vi "Extract subclasses from Pressure device.vi"(9 "Data In":string, 10 "Class":string, 11 "Pressure Device Settings in":T1) -> (1 "Data out":string, 3 "Pressure Device Settings out":T1)   [LabVIEW 2014, in "Mercury iXX.lvlib" / "Pressure.lvlib"]
uses:
  Pressure.lvlib
  Program Files (x86)/National Instruments/LabVIEW 2014/Public/Libraries/Pressure/Controls/Pressure Device (Read).ctl
  Controls/Manufacturing Data.ctl
  Controls/Pressure Sensor Type.ctl
  Controls/Calibration Cluster.ctl
  Controls/Calibration Interpolation.ctl
  Controls/Loop Cluster.ctl
  Controls/Pressure Signals Cluster.ctl
  Mercury iXX.lvlib
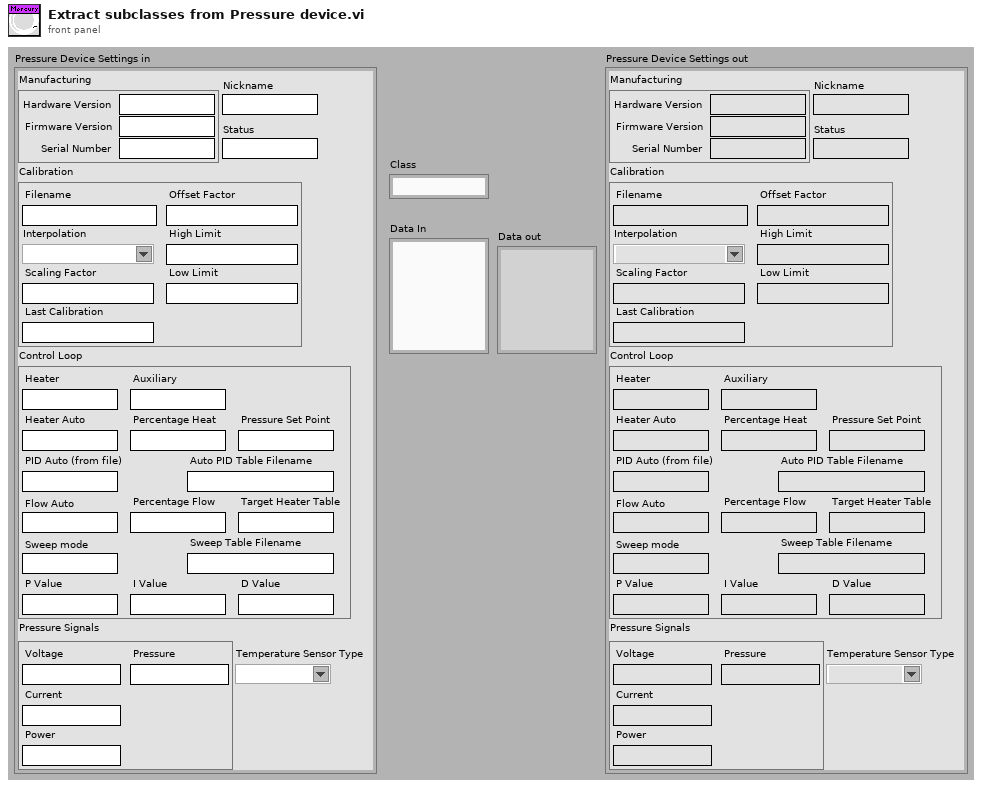
[diagram p1: front panel]
types:
  T1 = typedef "Mercury iXX.lvlib/Pressure.lvlib/Pressure Device (Read).ctl" = cluster{"Manufacturing":T2, "Temperature Sensor Type":T3, "Calibration":T4, "Control Loop":T6, "Pressure Signals":T7, "Nickname":string, "Status":string}
  T2 = typedef "Mercury iXX.lvlib/Manufacturing Data.ctl" = cluster{"Hardware Version":string, "Firmware Version":string, "Serial Number":string}
  T3 = typedef "Mercury iXX.lvlib/Pressure.lvlib/Pressure Sensor Type.ctl" = string
  T4 = typedef "Mercury iXX.lvlib/Pressure.lvlib/Calibration Cluster.ctl" = cluster{"Filename":string, "Interpolation":T5, "Scaling Factor":string, "Offset Factor":string, "High Limit":string, "Low Limit":string, "Last Calibration":string}
  T5 = typedef "Mercury iXX.lvlib/Pressure.lvlib/Calibration Interpolation.ctl" = string
  T6 = typedef "Mercury iXX.lvlib/Pressure.lvlib/Loop Cluster.ctl" = cluster{"Heater":string, "Auxiliary":string, "Heater Auto":string, "Percentage Heat":string, "Pressure Set Point":string, "PID Auto (from file)":string, "P Value":string, "I Value":string, "D Value":string, "Auto PID Table Filename":string, "Flow Auto":string, "Target Heater Table":string, "Sweep mode":string, "Sweep Table Filename":string, "Percentage Flow":string}
  T7 = typedef "Mercury iXX.lvlib/Pressure.lvlib/Pressure Signals Cluster.ctl" = cluster{"Voltage":string, "Current":string, "Power":string, "Pressure":string}
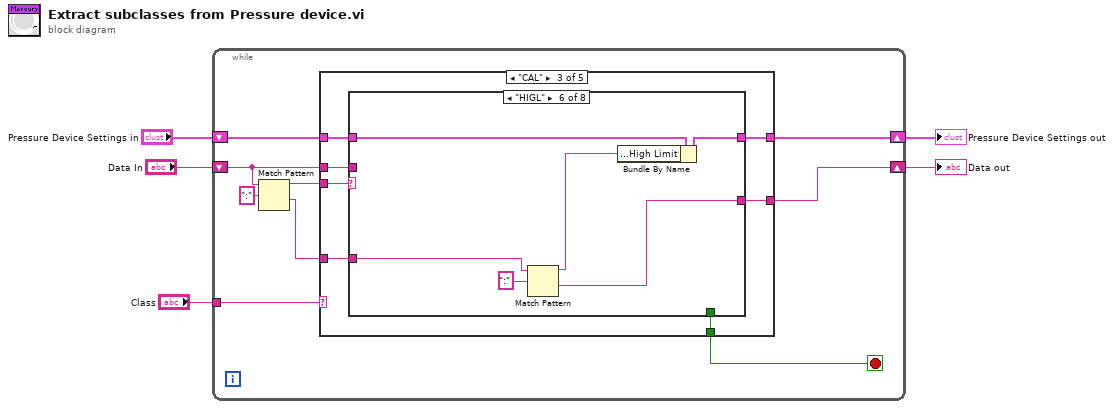
[diagram p0: block diagram]
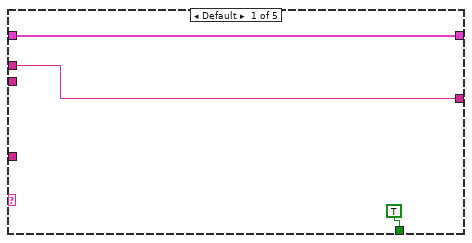
[diagram p2: hidden frame]
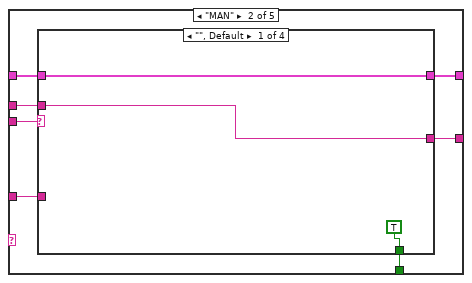
[diagram p3: hidden frame]
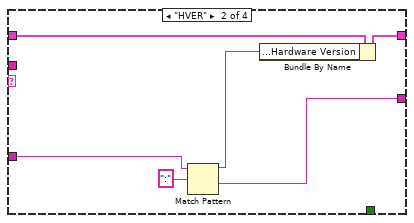
[diagram p4: hidden frame]
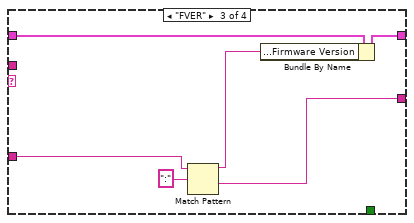
[diagram p5: hidden frame]
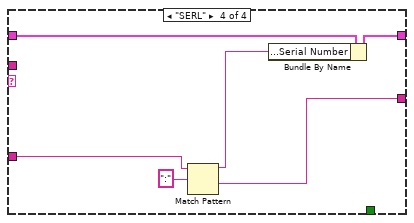
[diagram p6: hidden frame]
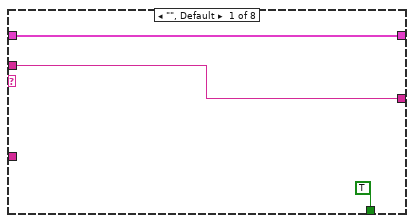
[diagram p7: hidden frame]
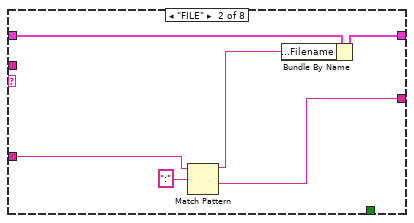
[diagram p8: hidden frame]
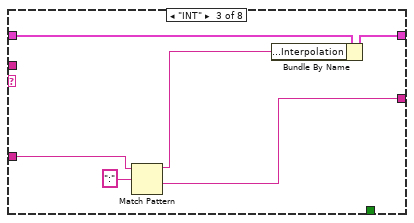
[diagram p9: hidden frame]
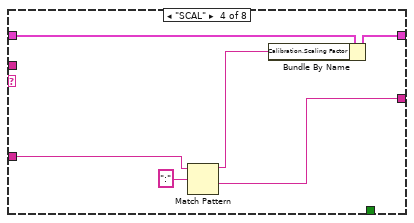
[diagram p10: hidden frame]
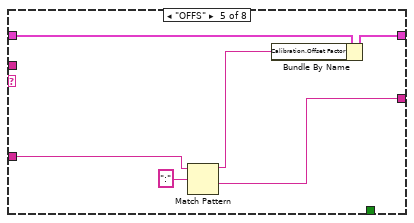
[diagram p11: hidden frame]
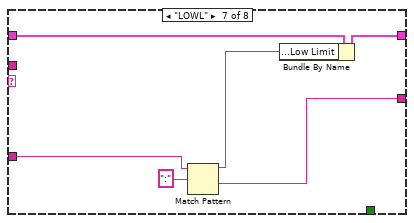
[diagram p12: hidden frame]
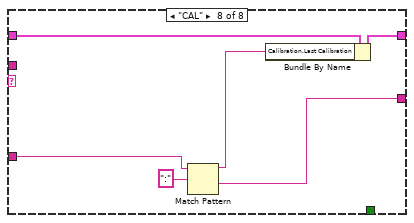
[diagram p13: hidden frame]
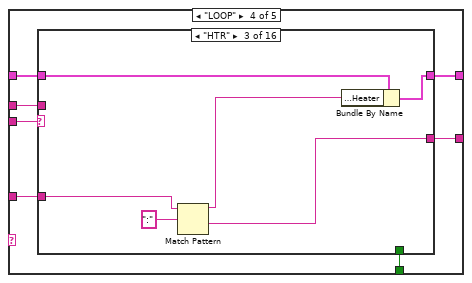
[diagram p14: hidden frame]
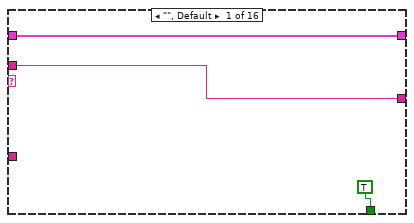
[diagram p15: hidden frame]
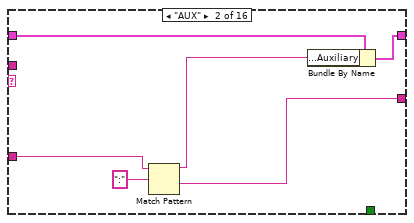
[diagram p16: hidden frame]
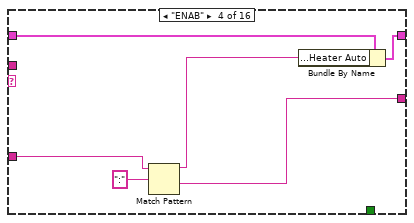
[diagram p17: hidden frame]
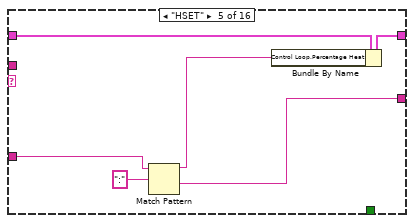
[diagram p18: hidden frame]
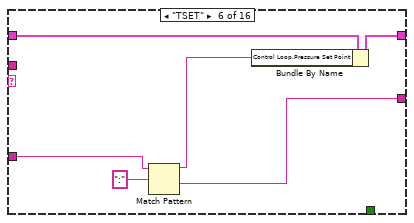
[diagram p19: hidden frame]
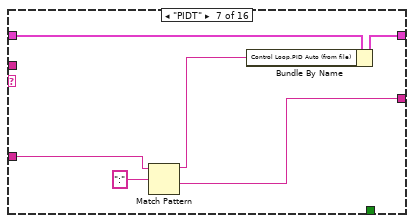
[diagram p20: hidden frame]
diagram:
  n1 = while {
    tunnel: "Class" -> [w7]
    shift-right: [w10] -> w4
    shift-left: "Data In" -> [w8]
    shift-right: [w12] -> w3
    shift-left: "Pressure Device Settings in" -> [w13]
    stop <- w6 stop-if-true
    n2 = Match Pattern(string=w8, regular expression=":") -> (before substring=w9:string, after substring=w11:string)  [unwired: 3 out]
    n3 = case shown="\"CAL\"" w7 {
      tunnel: w13 -> [w17 w24 w52 w104 w204]
      tunnel: [w17 w23 w51 w103 w203] -> w12
      tunnel: w11 -> [_ w22 w50 w102 w202]
      tunnel: [w16 w21 w49 w101 w201] -> w10
      tunnel: w9 -> [_ w20 w48 w100 w200]
      tunnel: w8 -> [w16 w19 w47 w99 w199]
      tunnel: [TRUE w18 w46 w98 w198] -> w6
      frame Default {
      }
      frame "MAN" {
        n4 = case shown="\"\", Default" w20 {
          tunnel: w24 -> [w27 w33 w39 w45]
          tunnel: [w27 w32 w38 w44] -> w23
          tunnel: w22 -> [_ w31 w37 w43]
          tunnel: [w26 w30 w36 w42] -> w21
          tunnel: w19 -> [w26 _ _ _]
          tunnel: [TRUE _ _ _] -> w18
          frame "", Default {
          }
          frame "HVER" {
            n5 = Match Pattern(string=w31, regular expression=":") -> (before substring=w28:string, after substring=w30:string)  [unwired: 3 out]
            n6 = Bundle By Name(cluster=w33, "Manufacturing.Hardware Version"=w28) -> (w32:T1)
          }
          frame "FVER" {
            n7 = Match Pattern(string=w37, regular expression=":") -> (before substring=w34:string, after substring=w36:string)  [unwired: 3 out]
            n8 = Bundle By Name(cluster=w39, "Manufacturing.Firmware Version"=w34) -> (w38:T1)
          }
          frame "SERL" {
            n9 = Match Pattern(string=w43, regular expression=":") -> (before substring=w40:string, after substring=w42:string)  [unwired: 3 out]
            n10 = Bundle By Name(cluster=w45, "Manufacturing.Serial Number"=w40) -> (w44:T1)
          }
        }
      }
      frame "CAL" {
        n11 = case shown="\"HIGL\"" w48 {
          tunnel: w52 -> [w55 w61 w67 w73 w79 w85 w91 w97]
          tunnel: [w55 w60 w66 w72 w78 w84 w90 w96] -> w51
          tunnel: w50 -> [_ w59 w65 w71 w77 w83 w89 w95]
          tunnel: [w54 w58 w64 w70 w76 w82 w88 w94] -> w49
          tunnel: w47 -> [w54 _ _ _ _ _ _ _]
          tunnel: [TRUE _ _ _ _ _ _ _] -> w46
          frame "", Default {
          }
          frame "FILE" {
            n12 = Match Pattern(string=w59, regular expression=":") -> (before substring=w56:string, after substring=w58:string)  [unwired: 3 out]
            n13 = Bundle By Name(cluster=w61, "Calibration.Filename"=w56) -> (w60:T1)
          }
          frame "INT" {
            n14 = Match Pattern(string=w65, regular expression=":") -> (before substring=w62:string, after substring=w64:string)  [unwired: 3 out]
            n15 = Bundle By Name(cluster=w67, "Calibration.Interpolation"=w62) -> (w66:T1)
          }
          frame "SCAL" {
            n16 = Match Pattern(string=w71, regular expression=":") -> (before substring=w68:string, after substring=w70:string)  [unwired: 3 out]
            n17 = Bundle By Name(cluster=w73, "Calibration.Scaling Factor"=w68) -> (w72:T1)
          }
          frame "OFFS" {
            n18 = Match Pattern(string=w77, regular expression=":") -> (before substring=w74:string, after substring=w76:string)  [unwired: 3 out]
            n19 = Bundle By Name(cluster=w79, "Calibration.Offset Factor"=w74) -> (w78:T1)
          }
          frame "HIGL" {
            n20 = Match Pattern(string=w83, regular expression=":") -> (before substring=w80:string, after substring=w82:string)  [unwired: 3 out]
            n21 = Bundle By Name(cluster=w85, "Calibration.High Limit"=w80) -> (w84:T1)
          }
          frame "LOWL" {
            n22 = Match Pattern(string=w89, regular expression=":") -> (before substring=w86:string, after substring=w88:string)  [unwired: 3 out]
            n23 = Bundle By Name(cluster=w91, "Calibration.Low Limit"=w86) -> (w90:T1)
          }
          frame "CAL" {
            n24 = Match Pattern(string=w95, regular expression=":") -> (before substring=w92:string, after substring=w94:string)  [unwired: 3 out]
            n25 = Bundle By Name(cluster=w97, "Calibration.Last Calibration"=w92) -> (w96:T1)
          }
        }
      }
      frame "LOOP" {
        n26 = case shown="\"HTR\"" w100 {
          tunnel: w104 -> [w107 w113 w119 w125 w131 w137 w143 w149 w155 w161 w167 w173 w179 w185 w191 w197]
          tunnel: [w107 w112 w118 w124 w130 w136 w142 w148 w154 w160 w166 w172 w178 w184 w190 w196] -> w103
          tunnel: w102 -> [_ w110 w116 w122 w128 w134 w140 w146 w153 w159 w165 w171 w177 w183 w189 w195]
          tunnel: [w106 w109 w115 w121 w127 w133 w139 w145 w152 w158 w164 w170 w176 w182 w188 w194] -> w101
          tunnel: w99 -> [w106 _ _ _ _ _ _ _ _ _ _ _ _ _ _ _]
          tunnel: [TRUE _ _ _ _ _ _ _ _ _ _ _ _ _ _ _] -> w98
          frame "", Default {
          }
          frame "AUX" {
            n27 = Match Pattern(string=w110, regular expression=":") -> (before substring=w108:string, after substring=w109:string)  [unwired: 3 out]
            n28 = Bundle By Name(cluster=w113, "Control Loop.Auxiliary"=w108) -> (w112:T1)
          }
          frame "HTR" {
            n29 = Match Pattern(string=w116, regular expression=":") -> (before substring=w114:string, after substring=w115:string)  [unwired: 3 out]
            n30 = Bundle By Name(cluster=w119, "Control Loop.Heater"=w114) -> (w118:T1)
          }
          frame "ENAB" {
            n31 = Match Pattern(string=w122, regular expression=":") -> (before substring=w120:string, after substring=w121:string)  [unwired: 3 out]
            n32 = Bundle By Name(cluster=w125, "Control Loop.Heater Auto"=w120) -> (w124:T1)
          }
          frame "HSET" {
            n33 = Match Pattern(string=w128, regular expression=":") -> (before substring=w126:string, after substring=w127:string)  [unwired: 3 out]
            n34 = Bundle By Name(cluster=w131, "Control Loop.Percentage Heat"=w126) -> (w130:T1)
          }
          frame "TSET" {
            n35 = Match Pattern(string=w134, regular expression=":") -> (before substring=w132:string, after substring=w133:string)  [unwired: 3 out]
            n36 = Bundle By Name(cluster=w137, "Control Loop.Pressure Set Point"=w132) -> (w136:T1)
          }
          frame "PIDT" {
            n37 = Match Pattern(string=w140, regular expression=":") -> (before substring=w138:string, after substring=w139:string)  [unwired: 3 out]
            n38 = Bundle By Name(cluster=w143, "Control Loop.PID Auto (from file)"=w138) -> (w142:T1)
          }
          frame "PIDF" {
            n39 = Match Pattern(string=w146, regular expression=":") -> (before substring=w144:string, after substring=w145:string)  [unwired: 3 out]
            n40 = Bundle By Name(cluster=w149, "Control Loop.Auto PID Table Filename"=w144) -> (w148:T1)
          }
          frame "P" {
            n41 = Match Pattern(string=w153, regular expression=":") -> (before substring=w150:string, after substring=w152:string)  [unwired: 3 out]
            n42 = Bundle By Name(cluster=w155, "Control Loop.P Value"=w150) -> (w154:T1)
          }
          frame "I" {
            n43 = Match Pattern(string=w159, regular expression=":") -> (before substring=w156:string, after substring=w158:string)  [unwired: 3 out]
            n44 = Bundle By Name(cluster=w161, "Control Loop.I Value"=w156) -> (w160:T1)
          }
          frame "D" {
            n45 = Match Pattern(string=w165, regular expression=":") -> (before substring=w162:string, after substring=w164:string)  [unwired: 3 out]
            n46 = Bundle By Name(cluster=w167, "Control Loop.D Value"=w162) -> (w166:T1)
          }
          frame "FAUT" {
            n47 = Match Pattern(string=w171, regular expression=":") -> (before substring=w168:string, after substring=w170:string)  [unwired: 3 out]
            n48 = Bundle By Name(cluster=w173, "Control Loop.Flow Auto"=w168) -> (w172:T1)
          }
          frame "FSET" {
            n49 = Match Pattern(string=w177, regular expression=":") -> (before substring=w174:string, after substring=w176:string)  [unwired: 3 out]
            n50 = Bundle By Name(cluster=w179, "Control Loop.Percentage Flow"=w174) -> (w178:T1)
          }
          frame "THTF" {
            n51 = Match Pattern(string=w183, regular expression=":") -> (before substring=w180:string, after substring=w182:string)  [unwired: 3 out]
            n52 = Bundle By Name(cluster=w185, "Control Loop.Target Heater Table"=w180) -> (w184:T1)
          }
          frame "SWMD" {
            n53 = Match Pattern(string=w189, regular expression=":") -> (before substring=w186:string, after substring=w188:string)  [unwired: 3 out]
            n54 = Bundle By Name(cluster=w191, "Control Loop.Sweep mode"=w186) -> (w190:T1)
          }
          frame "SWFL" {
            n55 = Match Pattern(string=w195, regular expression=":") -> (before substring=w192:string, after substring=w194:string)  [unwired: 3 out]
            n56 = Bundle By Name(cluster=w197, "Control Loop.Sweep Table Filename"=w192) -> (w196:T1)
          }
        }
      }
      frame "SIG" {
        n57 = case shown="\"PRES\"" w200 {
          tunnel: w204 -> [w207 w213 w219 w225 w231]
          tunnel: [w207 w212 w218 w224 w230] -> w203
          tunnel: w202 -> [_ w211 w217 w223 w229]
          tunnel: [w206 w210 w216 w222 w228] -> w201
          tunnel: w199 -> [w206 _ _ _ _]
          tunnel: [TRUE _ _ _ _] -> w198
          frame "", Default {
          }
          frame "VOLT" {
            n58 = Match Pattern(string=w211, regular expression=":") -> (before substring=w208:string, after substring=w210:string)  [unwired: 3 out]
            n59 = Bundle By Name(cluster=w213, "Pressure Signals.Voltage"=w208) -> (w212:T1)
          }
          frame "CURR" {
            n60 = Match Pattern(string=w217, regular expression=":") -> (before substring=w214:string, after substring=w216:string)  [unwired: 3 out]
            n61 = Bundle By Name(cluster=w219, "Pressure Signals.Current"=w214) -> (w218:T1)
          }
          frame "POWR" {
            n62 = Match Pattern(string=w223, regular expression=":") -> (before substring=w220:string, after substring=w222:string)  [unwired: 3 out]
            n63 = Bundle By Name(cluster=w225, "Pressure Signals.Power"=w220) -> (w224:T1)
          }
          frame "PRES" {
            n64 = Match Pattern(string=w229, regular expression=":") -> (before substring=w226:string, after substring=w228:string)  [unwired: 3 out]
            n65 = Bundle By Name(cluster=w231, "Pressure Signals.Pressure"=w226) -> (w230:T1)
          }
        }
      }
    }
  }
  "Data out" <- w4
  "Pressure Device Settings out" <- w3
